vi "Process.vi"(8 "error in":errorcluster, 11 "DAQ":refnum<class "DAQ.lvclass">) -> (0 "error out":errorcluster, 3 "DAQ out":refnum<class "DAQ.lvclass">)   [LabVIEW 2019, in "DAQ.lvclass"]
doc: "---------------------------------------------------------------\nJKI State Machine Objects™\nhttp://jki.net/state-machine-objects/\nCopyright (C) 2005-2015, JKI <info@jki.net>\nALL RIGHTS RESERVED"
uses:
  DAQ.lvclass
  <vilib>/JKI/JKI SMO/SMO/SMO.lvclass
  <vilib>/JKI/JKI SMO/SMO/Typedefs/Parent Call--Enum.ctl
  Typedefs/PrivateEvents--DAQ.SetWaveform.ctl
  C:/Program Files (x86)/National Instruments/LabVIEW 2016/vi.lib/JKI/JKI SMO/SMO/SMO.lvclass
panel:
  out "Name":string
  # "DAQ process.vi"
  # "For instructions on how to use the JKI State Machine Objects, examples and video tutorials, visit:\nhttp://jki.net/state-machine-objects/\n\nJKI State Machine Objects™\nhttp://jki.net/state-machine-objects/\nCopyright (C) 2005-2015, JKI <info@jki.net>\nALL RIGHTS RESERVED"
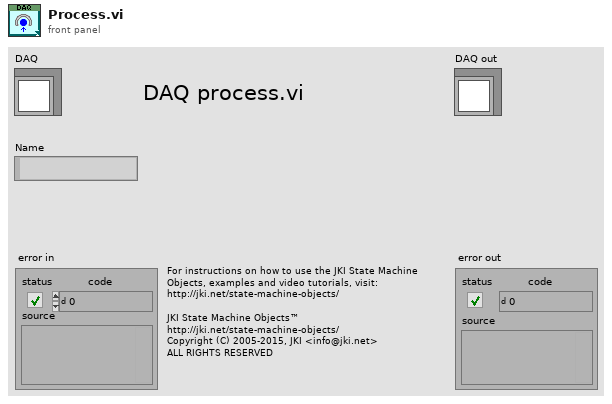
[diagram p1: front panel]
types:
  T1 = typedef "SMO.lvclass/Parent Call--Enum.ctl" = enum16{"Allows parent to run", "Does not request parent to run"}
  T2 = enum32{"invalid app kind", "Development System", "Run Time System", "Student Edition", "Embedded LabVIEW", "Evaluation", "Custom"}
  T3 = enum32{"Invalid", "Standard", "Closed", "Hidden", "Minimized", "Maximized"}
  T4 = enum32{"Bad", "Idle", "Run top level", "Running"}
  T5 = typedef "DAQ.lvclass/DAQ_Type.ctl" = enum16{"AI", "AO"}
  T6 = typedef "DAQ.lvclass/DAQ_SamplingInfo.ctl" = cluster{"Fs":dbl, "#s":i32}
  T7 = typedef "DAQ.lvclass/PrivateEvents--DAQ.SetWaveform.ctl" = waveform(dbl)[]
  T8 = cluster{"Core":cluster{"Current VI Reference":refnum<vi>, "Close Panel on Exit?":bool, "error":errorcluster}, "Self Reference":refnum<class "DAQ.lvclass">, "Channels":string, "DAQ_Type":T5, "DAQ_SamplingInfo":T6, "SetWaveform":T7, "to":i32}
  T9 = cluster{"Current VI Reference":refnum<vi>, "Close Panel on Exit?":bool, "error":errorcluster}
  T10 = typedef "SMO.lvclass/Protected Events.ctl" = cluster{"StopProcesses":refnum<user-event>, "AbortProcesses":refnum<user-event>, "Config Changed":refnum<user-event>, "Dependency":refnum<user-event>}
  T11 = typedef "DAQ.lvclass/PrivateEvents--Cluster.ctl" = cluster{"DAQ.Write":refnum<user-event>, "DAQ.setWaveform":refnum<user-event>}
  T12 = typedef "DAQ.lvclass/PrivateEvents--DAQ.Write.ctl" = waveform(dbl)[]
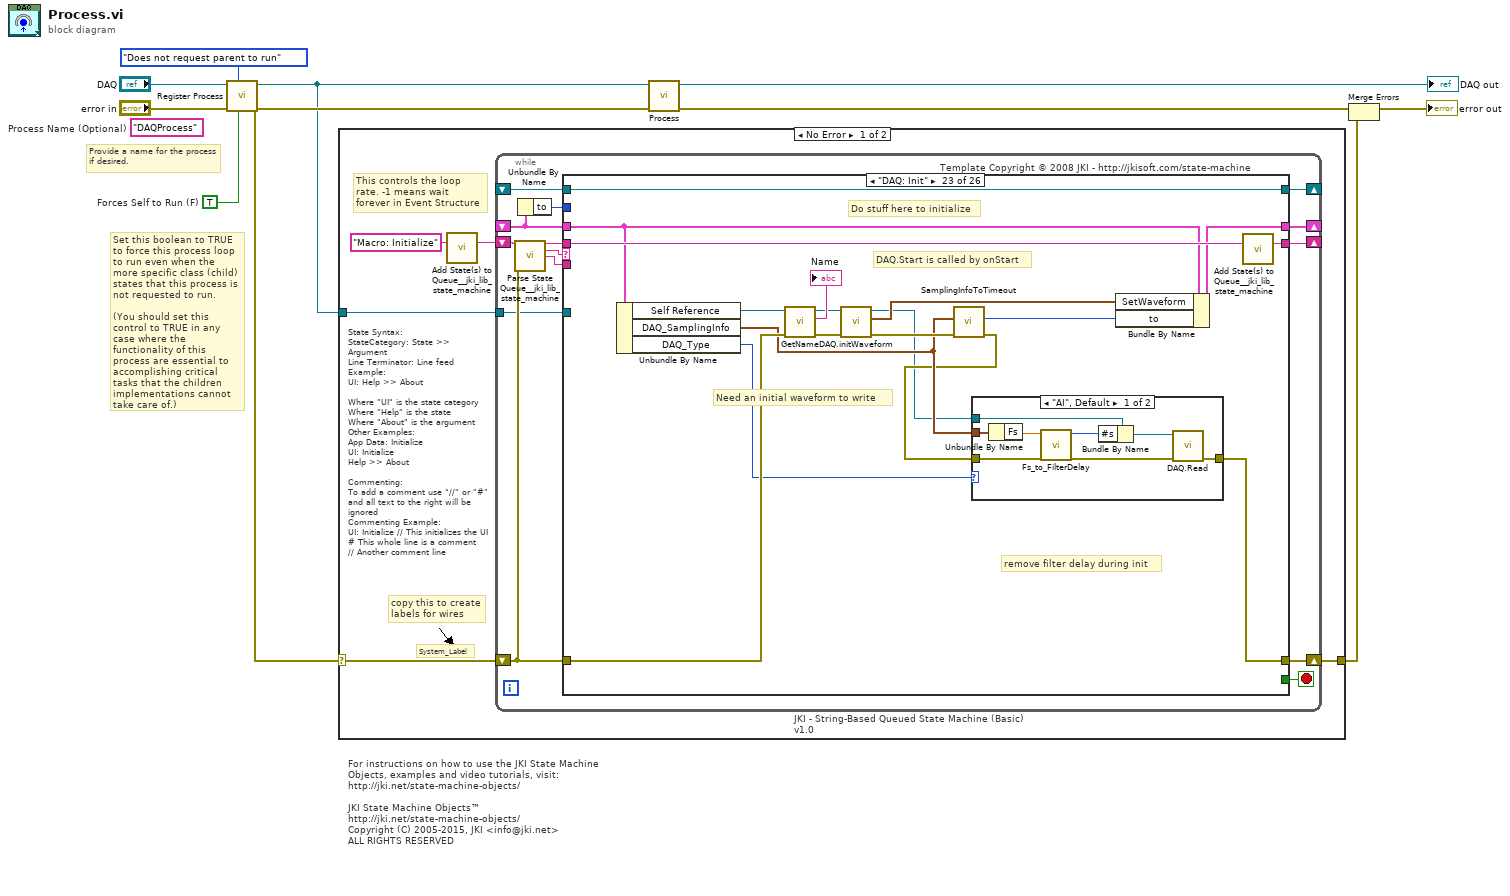
[diagram p0: block diagram]
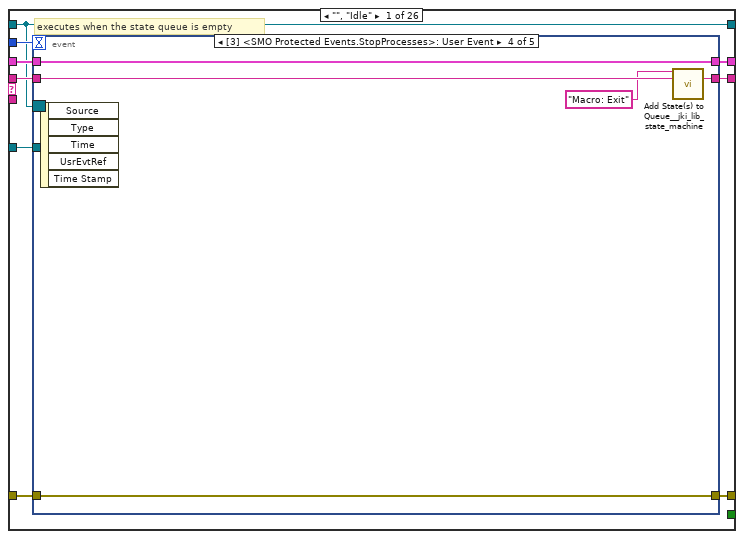
[diagram p2: hidden frame]
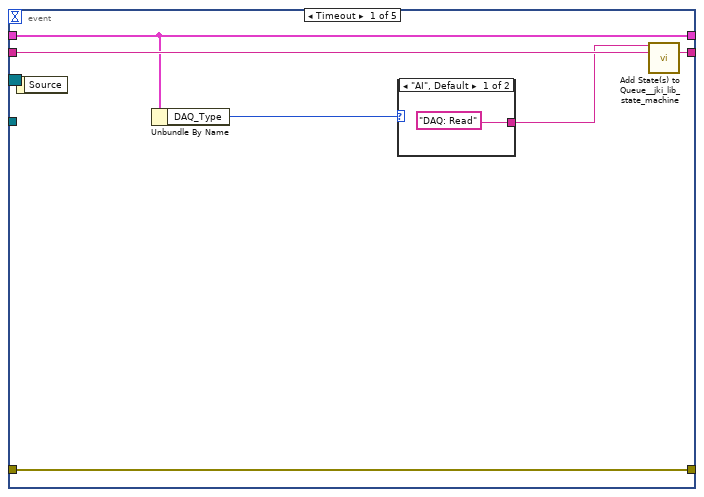
[diagram p3: hidden frame]
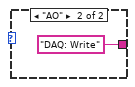
[diagram p4: hidden frame]
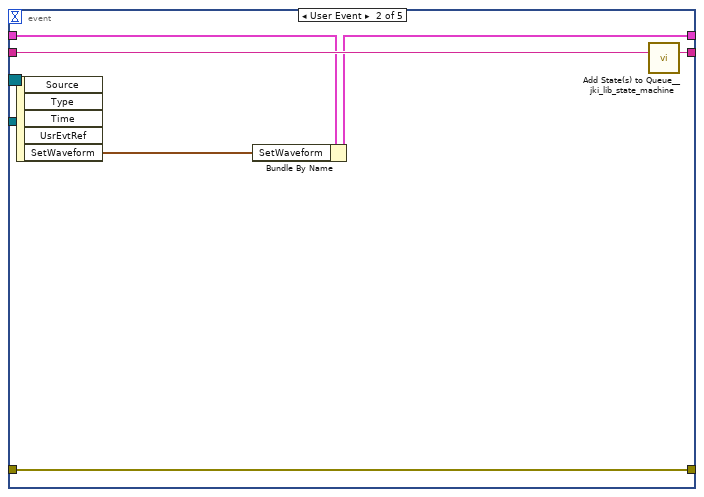
[diagram p5: hidden frame]
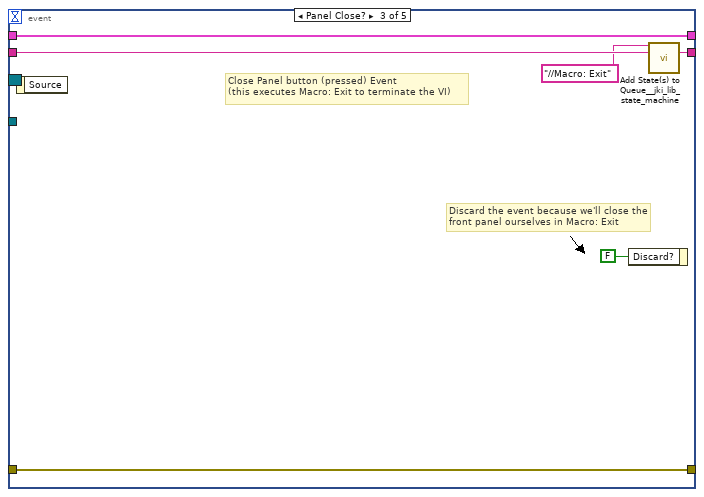
[diagram p6: hidden frame]
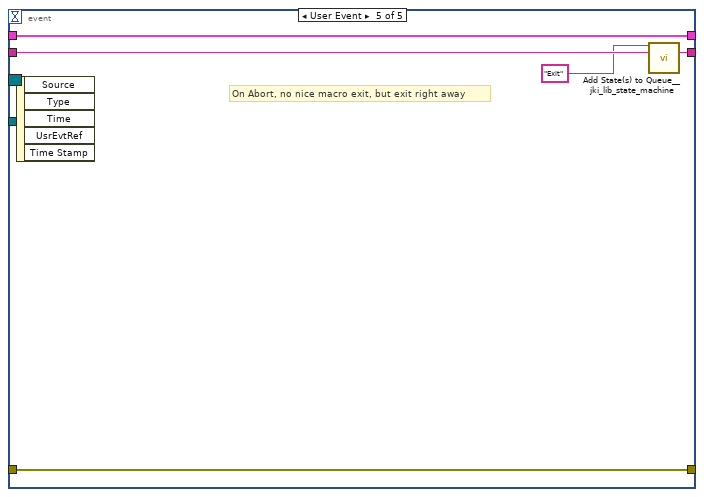
[diagram p7: hidden frame]
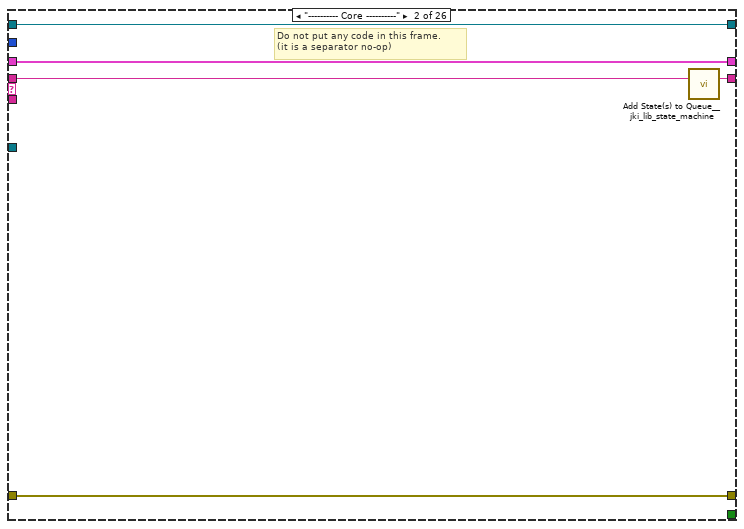
[diagram p8: hidden frame]
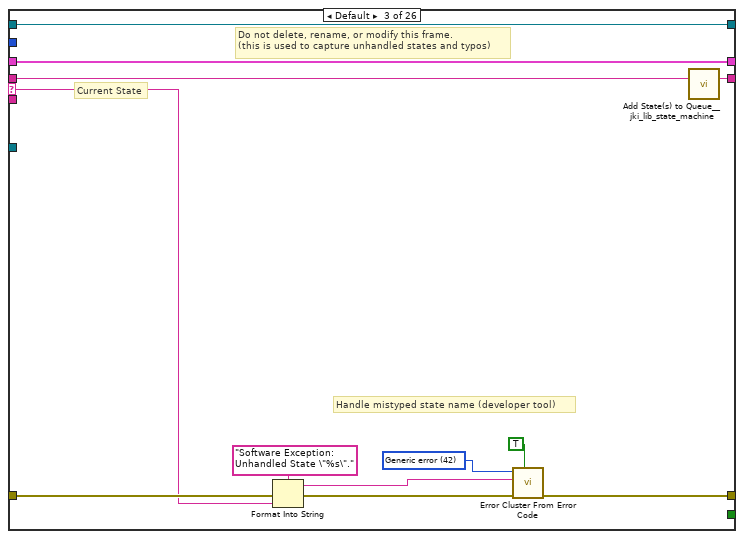
[diagram p9: hidden frame]
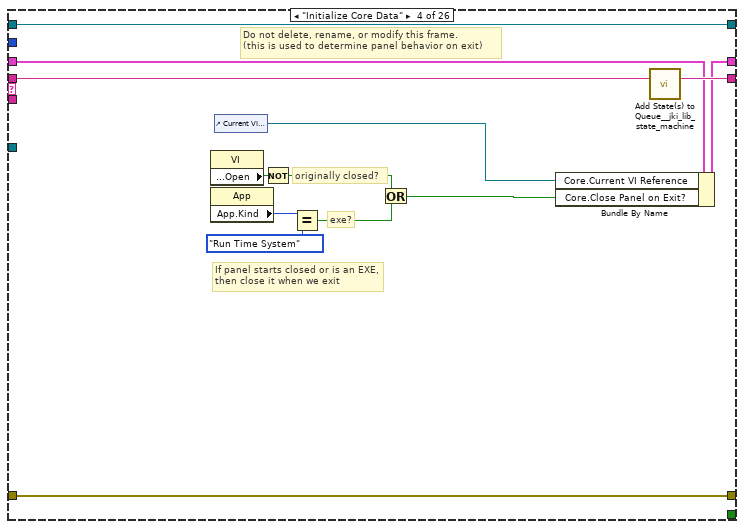
[diagram p10: hidden frame]
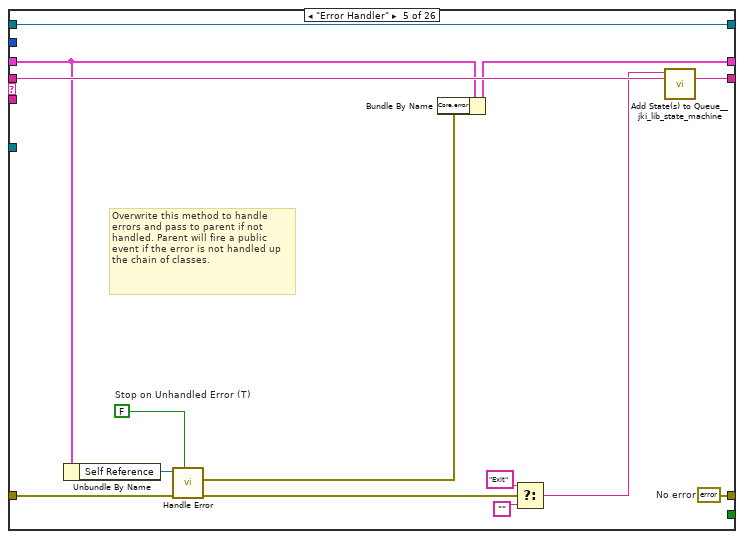
[diagram p11: hidden frame]
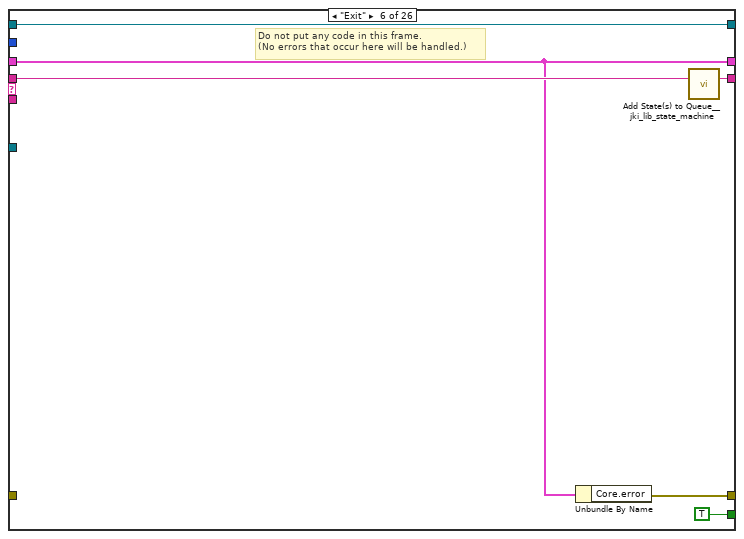
[diagram p12: hidden frame]
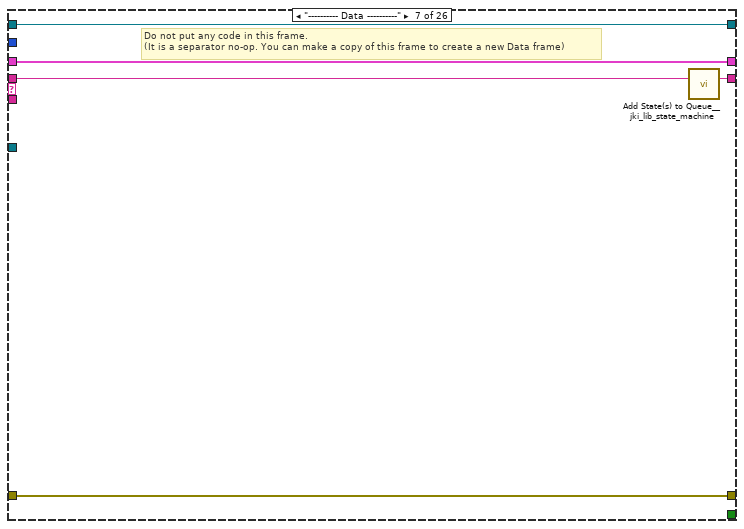
[diagram p13: hidden frame]
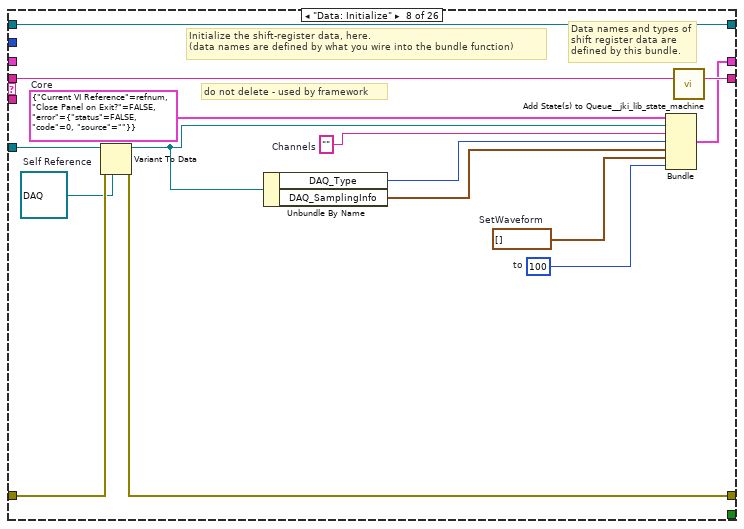
[diagram p14: hidden frame]
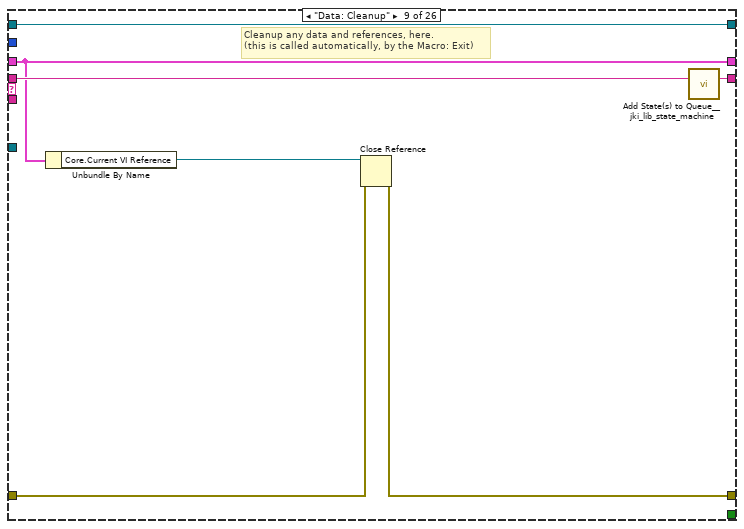
[diagram p15: hidden frame]
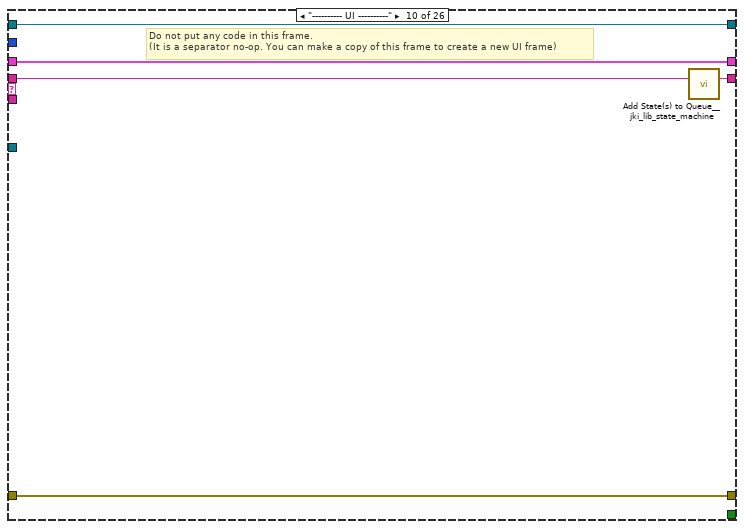
[diagram p16: hidden frame]
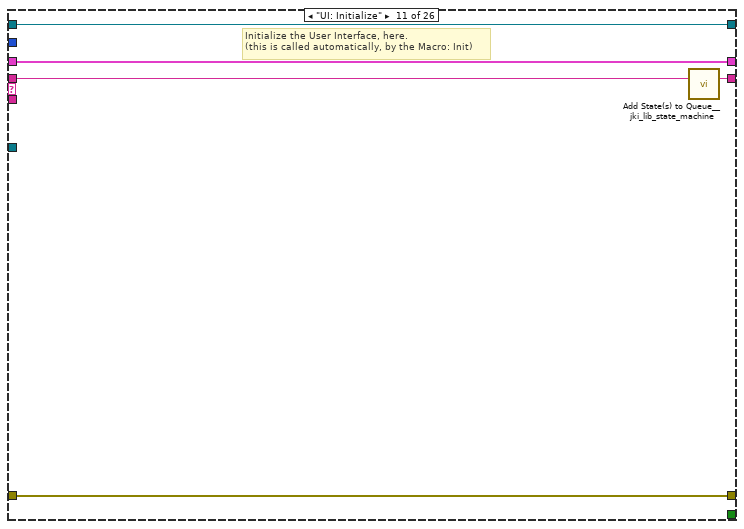
[diagram p17: hidden frame]
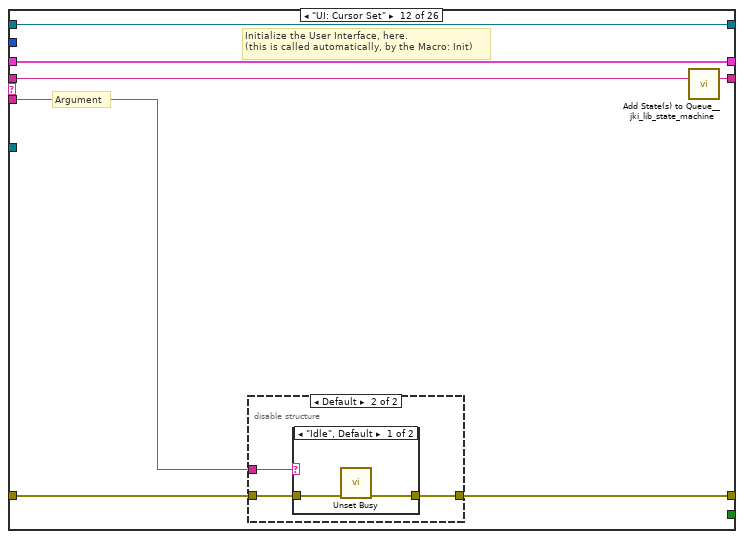
[diagram p18: hidden frame]
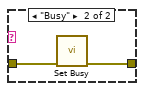
[diagram p20: hidden frame]
diagram:
  w1 = TRUE  # Forces Self to Run (F)
  (unwired) "DAQProcess"  # Process Name (Optional)
  # "Provide a name for the process\nif desired."
  # "Set this boolean to TRUE to force this process loop to run even when the more specific class (child) states that this process is not requested to run.\n\n(You should set this control to TRUE in any case where the functionality of this process are essential to accomplishing critical tasks that the children implementations cannot take care of.)"
  # "For instructions on how to use the JKI State Machine Objects, examples and video tutorials, visit:\nhttp://jki.net/state-machine-objects/\n\nJKI State Machine Objects™\nhttp://jki.net/state-machine-objects/\nCopyright (C) 2005-2015, JKI <info@jki.net>\nALL RIGHTS RESERVED"
  n1 = call <vilib>:"Register Process.vi"("Forces Self to Run (F)"=w1, "Parent Call"=Parent_Call--Enum."Does not request parent to run", "error in (no error)"="error in", "SMO"="DAQ") -> ("error out"=w7:errorcluster, "SMO out"=w6:refnum<class "DAQ.lvclass">)  [unwired: 6 in]
  n2 = case shown="No Error" w7 {
    selector: w7 -> [w12 w338]
    tunnel: w6 -> [w13 _]
    tunnel: [w11 w338] -> w3
    frame No Error {
      # "State Syntax:\nStateCategory: State >> Argument\nLine Terminator: Line feed\nExample:\nUI: Help >> About\n\nWhere \"UI\" is the state category\nWhere \"Help\" is the state\nWhere \"About\" is the argument\nOther Examples:\nApp Data: Initialize\nUI: Initialize\nHelp >> About\n\nCommenting:\nTo add a comment use \"//\" or \"#\" and all text to the right will be ignored\nCommenting Example:\nUI: Initialize // This initializes the UI\n# This whole line is a comment\n// Another comment line"
      # "copy this to create labels for wires"
      # "This controls the loop rate. -1 means wait forever in Event Structure"
      # "System_Label"
      n3 = call <vilib>:"Add State(s) to Queue__jki_lib_state_machine.vi"("State(s) in (\"\")"="Macro: Initialize") -> ("States Out"=w15:string)  [unwired: 14 in]
      n4 = while "JKI - String-Based Queued State Machine (Basic) v1.0" {
        shift-right: [w23] -> _
        shift-left: _ -> [w16]
        shift-right: [w18] -> w11
        shift-left: w12 -> [w22]
        shift-right: [w25] -> _
        shift-left: w15 -> [w26]
        tunnel: w13 -> [w21]
        shift-right: [w20] -> _
        shift-left: _ -> [w19]
        stop <- w24 stop-if-true
        # "Template Copyright © 2008 JKI - http://jkisoft.com/state-machine"
        n5 = call <vilib>:"Parse State Queue__jki_lib_state_machine.vi"("State Queue"=w26, "Error In (no error)"=w22) -> ("Remaining States"=w28:string, "Current State"=w29:string, "Arguments"=w27:string)  [unwired: 11 in]
        n6 = Unbundle By Name(w16) -> ("to"=w17:i32)
        n7 = case shown="\"DAQ: Init\"" w29 {
          selector: w29 -> [_ _ w75 _ _ _ _ _ _ _ _ _ _ _ _ _ _ _ _ _ _ _ _ _ _ _]
          tunnel: w28 -> [w38 w73 w79 w98 w112 w118 w123 w138 w145 w150 w155 w162 w180 w212 w226 w240 w245 w256 w261 w274 w280 w285 w303 w321 w332 w337]
          tunnel: w27 -> [_ _ _ _ _ _ _ _ _ _ _ w156 w175 _ _ _ _ _ _ _ _ _ _ _ _ _]
          tunnel: w16 -> [w36 w70 w77 w89 w106 w114 w120 _ w140 w147 w153 w160 w177 w209 w222 w231 w242 w253 w258 w272 w278 w283 w300 w312 w325 w333]
          tunnel: w22 -> [w34 w71 w80 w95 w108 _ w121 w134 w142 w148 w152 w158 w178 w210 w224 w238 w243 w248 w259 w268 w276 w281 w294 w314 w326 w334]
          tunnel: [w37 w72 w78 w97 w111 w117 w122 w137 w144 w149 w154 w161 w179 w211 w225 w239 w244 w255 w260 w273 w279 w284 w302 w320 w331 w336] -> w25
          tunnel: [_ _ _ _ _ TRUE _ _ _ _ _ _ _ _ _ _ _ _ _ _ _ _ _ _ _ _] -> w24
          tunnel: [w33 w70 w77 w96 w105 w114 w120 w136 w140 w147 w153 w160 w177 w209 w222 w231 w242 w253 w258 w272 w278 w283 w299 w312 w325 w333] -> w23
          tunnel: w17 -> [w32 _ _ _ _ _ _ _ _ _ _ _ _ _ _ _ _ _ _ _ _ _ _ _ _ _]
          tunnel: w21 -> [w30 _ _ _ _ _ _ w131 _ _ _ _ _ _ _ _ _ _ _ _ _ _ _ _ _ _]
          tunnel: [w31 w69 w74 w86 w110 w115 w119 w130 w139 w146 w151 w159 w174 w208 w223 w232 w241 w254 w257 w271 w277 w282 w301 w319 w330 w335] -> w20
          tunnel: w19 -> [w31 w69 w74 w86 w110 w115 w119 w130 w139 w146 w151 w159 w174 w208 w223 w232 w241 w254 w257 _ w277 w282 w301 w319 w330 w335]
          tunnel: [w35 w71 w81 w95 w107 w113 w121 w133 w141 w148 w152 w157 w172 w210 w224 w238 w243 w247 w259 w267 w276 w281 w286 w313 w324 w334] -> w18
          frame "", "Idle" {
            # "executes when the state queue is empty"
            n8 = event shown="[3] <SMO Protected Events.StopProcesses>: User Event" {
              selector: w31 -> [_ _ _ _ _]
              dyn-events: _ -> [_ _ _ _ _]
              timeout: w32 -> [_ _ _ _ _]
              tunnel: w38 -> [w44 w52 w58 w63 w68]
              tunnel: [w43 w51 w57 w62 w67] -> w37
              tunnel: w36 -> [w41 w49 w55 w60 w65]
              tunnel: [w42 w50 w56 w61 w66] -> w35
              tunnel: w34 -> [w42 w50 w56 w61 w66]
              tunnel: [w41 w48 w55 w60 w65] -> w33
              tunnel: w30 -> [_ _ _ _ _]
              event Timeout {
                n9 = event-data() -> ()  [unwired: 1 in, 1 out]
                n10 = Unbundle By Name(w41) -> ("DAQ_Type"=w40:T5)
                n11 = case shown="\"AI\", Default" w40 {
                  tunnel: ["DAQ: Read" ("State(s) at Back (\"\")") "DAQ: Write" ("State(s) at Back (\"\")")] -> w39
                  frame "AI", Default {
                  }
                  frame "AO" {
                  }
                }
                n12 = call <vilib>:"Add State(s) to Queue__jki_lib_state_machine.vi"("State(s) in Front (\"\")"=w39, "State(s) in (\"\")"=w44) -> ("States Out"=w43:string)  [unwired: 13 in]
              }
              event User Event {
                n13 = event-data() -> ("SetWaveform"=w47:waveform(dbl)[])  [unwired: 1 in, 4 out]
                n14 = Bundle By Name(cluster=w49, "SetWaveform"=w47) -> (w48:T8)
                n15 = call <vilib>:"Add State(s) to Queue__jki_lib_state_machine.vi"("State(s) in (\"\")"=w52) -> ("States Out"=w51:string)  [unwired: 14 in]
              }
              event Panel Close? {
                # "Discard the event because we'll close the front panel ourselves in Macro: Exit"
                # "Close Panel button (pressed) Event\n(this executes Macro: Exit to terminate the VI)"
                n16 = event-data() -> ()  [unwired: 1 in, 1 out]
                n17 = event-data("Discard?"=FALSE) -> ()  [unwired: 1 in, 1 out]
                n18 = call <vilib>:"Add State(s) to Queue__jki_lib_state_machine.vi"("State(s) in Front (\"\")"="//Macro: Exit", "State(s) in (\"\")"=w58) -> ("States Out"=w57:string)  [unwired: 13 in]
              }
              event User Event {
                n19 = event-data() -> ()  [unwired: 1 in, 5 out]
                n20 = call <vilib>:"Add State(s) to Queue__jki_lib_state_machine.vi"("State(s) in Front (\"\")"="Macro: Exit", "State(s) in (\"\")"=w63) -> ("States Out"=w62:string)  [unwired: 13 in]
              }
              event User Event {
                # "On Abort, no nice macro exit, but exit right away"
                n21 = event-data() -> ()  [unwired: 1 in, 5 out]
                n22 = call <vilib>:"Add State(s) to Queue__jki_lib_state_machine.vi"("State(s) in Front (\"\")"="Exit", "State(s) in (\"\")"=w68) -> ("States Out"=w67:string)  [unwired: 13 in]
              }
            }
          }
          frame "---------- Core ----------" {
            # "Do not put any code in this frame.\n(it is a separator no-op)"
            n23 = call <vilib>:"Add State(s) to Queue__jki_lib_state_machine.vi"("State(s) in (\"\")"=w73) -> ("States Out"=w72:string)  [unwired: 14 in]
          }
          frame Default {
            w84 = 42 items=["No error", "Argument error", "Memory is full", "Out of zone", "End of file", "File already open", "Generic file I/O error", "File not found", "File permission error", "Disk is full", "Duplicate path", "Too many files open", "System feature not enabled", "Resource file not found", "Cannot add resource", "Resource not found", "Image not found", "Image memory error", "Pen does not exist", "Config type invalid", "Config token not found", "Config parse error", "Config memory error", "Bad external code format", "Bad external code offset", "External code not present", "Null window", "Destroy window error", "Null menu", "Print aborted", "Bad print record", "Print driver error", "Windows error during printing", "Memory error during printing", "Print dialog error", "Generic print error", "Invalid device refnum", "Device not found", "Device parameter error", "Device unit error", "Cannot open device", "Device call aborted", "Generic error", "Cancelled by user", "Object ID too low", "Object ID too high", "Object not in heap", "Unknown heap", "Unknown object (invalid DefProc)", "Unknown object (DefProc not in table)", "Message out of range", "Invalid (null) method", "Unknown message", "Manager call not supported", "Bad address", "Network operation in progress", "Network operation timed out", "Connection is busy", "Network attribute not supported", "Network error", "Address in use", "System out of memory", "Connection aborted", "Connection refused", "Not connected", "Already connected", "Connection closed", "Initialization error (interapplication manager)", "Bad occurrence", "Wait on unbound occurrence handler", "Occurrence queue overflow", "Datalog type conflict", "Unused", "Unrecognized type (interapplication manager)", "Memory corrupt", "Failed to make temporary DLL", "Old CIN version", "Drag socket not found", "Failed to load drop-object", "Failed to register OLE object", "Failed to release OLE object", "Format specifier type mismatch", "Unknown format specifier", "Too few format specifiers", "Too many format specifiers", "Scan failed", "Newer CIN version", "Error converting to variant", "Runtime menu error", "Password tampered", "Variant attribute not found", "Incompatible variant data type", "Event data is not available", "Event Store is not present", "Occurrence is not found", "Event Queue is not created", "Event info is not available", "Refnum passed is NULL", "Error retrieving Class GUID", "Error retrieving CoClass GUID", "Error retrieving TypeLib GUID.", "Bad built application magic bytes.", "Specific driver is different from the specific driver associated with the Logical Name.", "There is no session opened to the class driver.", "Max Error", "MAX - Error with config objects", "MAX - Error loading configuration", "MAX - Group not supported"]
            # "Current State"
            # "Do not delete, rename, or modify this frame.\n(this is used to capture unhandled states and typos)"
            # "Handle mistyped state name (developer tool)"
            n24 = Format Into String(format string="Software Exception: Unhandled State \"%s\"." ("message"), error in=w80, w75) -> (resulting string=w83:string, error out=w82:errorcluster)  [unwired: 1 in]
            n25 = call <vilib>:"Error Cluster From Error Code.vi"("show call chain? (False)"=TRUE, "error in (no error)"=w82, "error message (\"\")"=w83, "error code (0)"=w84) -> ("error out"=w81:errorcluster)  [unwired: 5 in]
            n26 = call <vilib>:"Add State(s) to Queue__jki_lib_state_machine.vi"("State(s) in (\"\")"=w79) -> ("States Out"=w78:string)  [unwired: 14 in]
          }
          frame "Initialize Core Data" {
            # "Do not delete, rename, or modify this frame.\n(this is used to determine panel behavior on exit)"
            # "originally closed?"
            # "exe?"
            # "If panel starts closed or is an EXE, then close it when we exit"
            n27 = property class="VI"() -> ("Front Panel.Open"=w94:bool)  [unwired: 2 in, 2 out]
            n28 = property class="App"() -> ("App.Kind"=w93:T2)  [unwired: 2 in, 2 out]
            n29 = control-ref of="Current VI Reference"() -> (w87:refnum<vi>)
            n30 = Not(x=w94) -> (.not. x?=w91:bool)
            n31 = Equal?(x=w93, y=T2."Run Time System" ("Application:Kind")) -> (x = y?=w90:bool)
            n32 = Or(x=w91, y=w90) -> (x .or. y?=w88:bool)
            n33 = Bundle By Name(cluster=w89, "Core.Current VI Reference"=w87, "Core.Close Panel on Exit?"=w88) -> (w96:T8)
            n34 = call <vilib>:"Add State(s) to Queue__jki_lib_state_machine.vi"("State(s) in (\"\")"=w98) -> ("States Out"=w97:string)  [unwired: 14 in]
          }
          frame "Error Handler" {
            w99 = FALSE  # Stop on Unhandled Error (T)
            w107 = errorcluster {"status"=FALSE, "code"=0, "source"=""}  # No error
            # "Overwrite this method to handle errors and pass to parent if not handled. Parent will fire a public event if the error is not handled up the chain of classes."
            n35 = Unbundle By Name(w106) -> ("Self Reference"=w109:refnum<class "DAQ.lvclass">)
            n36 = call-dynamic "Handle Error.vi"("Stop on Unhandled Error (T)"=w99, "error in"=w108, "SMO"=w109) -> ("handling error"=w100:errorcluster, "Unhandled error"=w103:errorcluster)  [unwired: 6 in, 1 out]
            n37 = Bundle By Name(cluster=w106, "Core.error"=w103) -> (w105:T8)
            n38 = Select(t="Exit", s=w100, f="") -> (s? t:f=w104:string)
            n39 = call <vilib>:"Add State(s) to Queue__jki_lib_state_machine.vi"("State(s) in Front (\"\")"=w104, "State(s) in (\"\")"=w112) -> ("States Out"=w111:string)  [unwired: 13 in]
          }
          frame "Exit" {
            # "Do not put any code in this frame.\n(No errors that occur here will be handled.)"
            n40 = Unbundle By Name(w114) -> ("Core.error"=w113:errorcluster)
            n41 = call <vilib>:"Add State(s) to Queue__jki_lib_state_machine.vi"("State(s) in (\"\")"=w118) -> ("States Out"=w117:string)  [unwired: 14 in]
          }
          frame "---------- Data ----------" {
            # "Do not put any code in this frame.\n(It is a separator no-op. You can make a copy of this frame to create a new Data frame)"
            n42 = call <vilib>:"Add State(s) to Queue__jki_lib_state_machine.vi"("State(s) in (\"\")"=w123) -> ("States Out"=w122:string)  [unwired: 14 in]
          }
          frame "Data: Initialize" {
            w126 = 100  # to
            w125 = T7 []  # SetWaveform
            w129 = T9 {"Current VI Reference"=refnum, "Close Panel on Exit?"=FALSE, "error"={"status"=FALSE, "code"=0, "source"=""}}  # Core
            w132 = refnum<class "DAQ.lvclass"> refnum  # Self Reference
            w135 = ""  # Channels
            # "do not delete - used by framework"
            # "Data names and types of shift register data are defined by this bundle."
            # "Initialize the shift-register data, here.\n(data names are defined by what you wire into the bundle function)"
            n43 = Variant To Data(error in=w134, type=w132, Variant=w131) -> (data=w128:refnum<class "DAQ.lvclass">, error out=w133:errorcluster)
            n44 = Unbundle By Name(w128) -> ("DAQ_Type"=w127:T5, "DAQ_SamplingInfo"=w124:T6)
            n45 = Bundle("Core"=w129, "Self Reference"=w128, "Channels"=w135, "DAQ_Type"=w127, "DAQ_SamplingInfo"=w124, "SetWaveform"=w125, "to"=w126) -> (w136:T8)  [unwired: 1 in]
            n46 = call <vilib>:"Add State(s) to Queue__jki_lib_state_machine.vi"("State(s) in (\"\")"=w138) -> ("States Out"=w137:string)  [unwired: 14 in]
          }
          frame "Data: Cleanup" {
            # "Cleanup any data and references, here.\n(this is called automatically, by the Macro: Exit)"
            n47 = Unbundle By Name(w140) -> ("Core.Current VI Reference"=w143:refnum<vi>)
            n48 = Close Reference(reference=w143, error in (no error)=w142) -> (error out=w141:errorcluster)
            n49 = call <vilib>:"Add State(s) to Queue__jki_lib_state_machine.vi"("State(s) in (\"\")"=w145) -> ("States Out"=w144:string)  [unwired: 14 in]
          }
          frame "---------- UI ----------" {
            # "Do not put any code in this frame.\n(It is a separator no-op. You can make a copy of this frame to create a new UI frame)"
            n50 = call <vilib>:"Add State(s) to Queue__jki_lib_state_machine.vi"("State(s) in (\"\")"=w150) -> ("States Out"=w149:string)  [unwired: 14 in]
          }
          frame "UI: Initialize" {
            # "Initialize the User Interface, here.\n(this is called automatically, by the Macro: Init)"
            n51 = call <vilib>:"Add State(s) to Queue__jki_lib_state_machine.vi"("State(s) in (\"\")"=w155) -> ("States Out"=w154:string)  [unwired: 14 in]
          }
          frame "UI: Cursor Set" {
            # "Argument"
            # "Initialize the User Interface, here.\n(this is called automatically, by the Macro: Init)"
            n52 = disable-structure shown="Default" {
              disable-tunnel: w158 -> [w163 w166]
              disable-tunnel: [w163 w165] -> w157
              disable-tunnel: w156 -> [_ w164]
              frame condition #0 {
              }
              frame condition #1 (active) {
                n53 = case shown="\"Idle\", Default" w164 {
                  tunnel: w166 -> [w168 w170]
                  tunnel: [w167 w169] -> w165
                  frame "Idle", Default {
                    n54 = call <vilib>:"Unset Busy.vi"("error in (no error)"=w168) -> ("error out"=w167:errorcluster)  [unwired: 10 in]
                  }
                  frame "Busy" {
                    n55 = call <vilib>:"Set Busy.vi"("error in (no error)"=w170) -> ("error out"=w169:errorcluster)  [unwired: 9 in, 1 out]
                  }
                }
              }
            }
            n56 = call <vilib>:"Add State(s) to Queue__jki_lib_state_machine.vi"("State(s) in (\"\")"=w162) -> ("States Out"=w161:string)  [unwired: 14 in]
          }
          frame "UI: Front Panel State" {
            # "use for debugging"
            # "Argument"
            # "Set Front Panel Open or Closed\n(Usage: \"UI: Front Panel State >> Open|Close\")"
            n57 = Unbundle By Name(w177) -> ("Core.Current VI Reference"=w176:refnum<vi>)
            n58 = disable-structure shown="Default" {
              disable-tunnel: w178 -> [w184 w207]
              disable-tunnel: [w183 w207] -> w171
              disable-tunnel: w176 -> [w182 _]
              disable-tunnel: w175 -> [w181 _]
              frame condition #0 (active) {
                n59 = case shown="\"Close\"" w181 {
                  tunnel: w184 -> [w188 w201]
                  tunnel: [w190 w202] -> w183
                  tunnel: w182 -> [w189 w199]
                  frame "Open", Default {
                    n60 = property class="VI"(reference=w189, error in=w188) -> (reference out=w186:refnum<vi>, error out=w187:errorcluster, "FP.State"=w185:T3)
                    n61 = case shown="\"Closed\"" w185 {
                      tunnel: [w193 w196] -> w190
                      tunnel: w187 -> [w192 w196]
                      tunnel: w186 -> [w191 _]
                      frame "Closed" {
                        n62 = invoke class="VI" method="FP.Open"(reference=w191, error in=w192, "Activate"=TRUE, "State"=T3."Standard") -> (error out=w193:errorcluster)  [unwired: 1 in, 4 out]
                      }
                      frame Default {
                      }
                    }
                  }
                  frame "Close" {
                    n63 = property class="VI"(reference=w199, error in=w201) -> (reference out=w198:refnum<vi>, error out=w200:errorcluster, "FP.State"=w197:T3)
                    n64 = case shown="Default" w197 {
                      tunnel: [w203 w206] -> w202
                      tunnel: w200 -> [w203 w205]
                      tunnel: w198 -> [_ w204]
                      frame "Invalid", "Closed" {
                      }
                      frame Default {
                        n65 = invoke class="VI" method="FP.Close"(reference=w204, error in=w205) -> (error out=w206:errorcluster)  [unwired: 1 in, 2 out]
                      }
                    }
                  }
                }
              }
              frame condition #1 {
              }
            }
            n66 = call <userlib>:"Wait (ms)__ogtk.vi"("error in (no error)"=w171, "milliseconds to wait"=u32 0) -> ("error out"=w172:errorcluster)  [unwired: 8 in, 1 out]
            n67 = call <vilib>:"Add State(s) to Queue__jki_lib_state_machine.vi"("State(s) in (\"\")"=w180) -> ("States Out"=w179:string)  [unwired: 14 in]
          }
          frame "---------- Macro ----------" {
            # "Do not put any code in this frame.\n(It is a separator no-op. You can make a copy of this frame to create a new Macro frame)"
            n68 = call <vilib>:"Add State(s) to Queue__jki_lib_state_machine.vi"("State(s) in (\"\")"=w212) -> ("States Out"=w211:string)  [unwired: 14 in]
          }
          frame "Macro: Initialize" {
            w213 = "Process: Sync"
            w218 = "Data: Initialize\nInitialize Core Data\nUI: Initialize\nUI: Front Panel State >> Open\nEvents: Register"  # Data: Initialize Initialize Core Data UI: Initialize UI: Front Panel State >> Open Events: Register
            # "Initialization Macro\n(This is called once, when the VI starts)"
            n69 = control-ref of="This VI"() -> (w215:refnum<vi>)
            n70 = property class="VI"(reference=w215) -> ("Exec.State"=w214:T4)  [unwired: 1 in, 2 out]
            n71 = Equal?(x=w214, y=T4."Run top level") -> (x = y?=w220:bool)
            n72 = Select(t=w213, s=w220, f="") -> ()  [unwired: 1 out]
            n73 = call <vilib>:"Add State(s) to Queue__jki_lib_state_machine.vi"("State(s) in Front (\"\")"=w218, "State(s) in (\"\")"=w213, "State(s) at Back (\"\")"="DAQ: Init") -> ("States Out"=w216:string)  [unwired: 12 in]
            n74 = call <vilib>:"Add State(s) to Queue__jki_lib_state_machine.vi"("State(s) in Front (\"\")"=w216, "State(s) in (\"\")"=w226) -> ("States Out"=w225:string)  [unwired: 13 in]
          }
          frame "Macro: Exit" {
            # "Exit Macro\n(This is called once, when the VI exits)"
            n75 = Unbundle By Name(w231) -> ("Core.Close Panel on Exit?"=w237:bool)
            n76 = Select(t="DAQ: Stop\nUI: Front Panel State >> Close", s=w237, f="") -> (s? t:f=w234:string)
            n77 = call <vilib>:"Add State(s) to Queue__jki_lib_state_machine.vi"("State(s) in Front (\"\")"="Data: Cleanup\nEvents: Unregister", "State(s) in (\"\")"="Process: Sync", "State(s) at Back (\"\")"="Exit") -> ("States Out"=w228:string)  [unwired: 12 in]
            n78 = call <vilib>:"Add State(s) to Queue__jki_lib_state_machine.vi"("State(s) in (\"\")"=w234, "State(s) at Back (\"\")"=w228) -> ("States Out"=w233:string)  [unwired: 13 in]
            n79 = call <vilib>:"Add State(s) to Queue__jki_lib_state_machine.vi"("State(s) in Front (\"\")"=w233, "State(s) in (\"\")"=w240) -> ("States Out"=w239:string)  [unwired: 13 in]
          }
          frame "---------- Process ----------" {
            # "Template Separator\n(You can make a copy of, or modify, this frame)"
            n80 = call <vilib>:"Add State(s) to Queue__jki_lib_state_machine.vi"("State(s) in (\"\")"=w245) -> ("States Out"=w244:string)  [unwired: 14 in]
          }
          frame "Process: Sync" {
            n81 = Unbundle By Name(w253) -> ("Self Reference"=w249:refnum<class "DAQ.lvclass">)
            n82 = call <vilib>:"WaitOnProcessSync.vi"("error in (no error)"=w248, "SMO"=w249) -> ("error out"=w247:errorcluster, "Don't run?"=w252:bool)  [unwired: 7 in, 1 out]
            n83 = Select(t="Data: Cleanup\nEvents: Unregister\nExit", s=w252, f="") -> (s? t:f=w246:string)
            n84 = call <vilib>:"Add State(s) to Queue__jki_lib_state_machine.vi"("State(s) in Front (\"\")"=w246, "State(s) in (\"\")"=w256) -> ("States Out"=w255:string)  [unwired: 13 in]
          }
          frame "---------- Events ----------" {
            # "Template Separator\n(You can make a copy of, or modify, this frame)"
            n85 = call <vilib>:"Add State(s) to Queue__jki_lib_state_machine.vi"("State(s) in (\"\")"=w261) -> ("States Out"=w260:string)  [unwired: 14 in]
          }
          frame "Events: Register" {
            # "Expand to add\nmore events"
            n86 = Unbundle By Name(w272) -> ("Self Reference"=w269:refnum<class "DAQ.lvclass">)
            n87 = call <vilib>:"GetProtectedEvents.vi"("SMO"=w269) -> ("error out"=w265:errorcluster, "SMO Protected Events"=w270:T10, "SMO out"=w262:refnum<class "DAQ.lvclass">)  [unwired: 8 in]
            n88 = call "DAQ.GetPrivateEvents.vi"("DAQ"=w262) -> ("error out"=w264:errorcluster, "Private Events"=w263:T11)  [unwired: 8 in, 1 out]
            n89 = register-events(w270, w263) -> (reference out=w271:refnum<event-registration>, error out=w266:errorcluster)  [unwired: 2 in]
            n90 = Merge Errors(w268, w266, w265, w264) -> (w267:errorcluster)
            n91 = call <vilib>:"Add State(s) to Queue__jki_lib_state_machine.vi"("State(s) in (\"\")"=w274) -> ("States Out"=w273:string)  [unwired: 14 in]
          }
          frame "Events: Unregister" {
            n92 = Unregister For Events(event registration refnum=w277, error in=w276) -> (error out=w275:errorcluster)
            n93 = call <vilib>:"Clear Errors.vi"("error in (no error)"=w275) -> ()  [unwired: 5 in, 2 out]
            n94 = call <vilib>:"Add State(s) to Queue__jki_lib_state_machine.vi"("State(s) in (\"\")"=w280) -> ("States Out"=w279:string)  [unwired: 14 in]
          }
          frame "---------- Action ----------" {
            n95 = call <vilib>:"Add State(s) to Queue__jki_lib_state_machine.vi"("State(s) in (\"\")"=w285) -> ("States Out"=w284:string)  [unwired: 14 in]
          }
          frame "DAQ: Init" {
            # "remove filter delay during init"
            # "Need an initial waveform to write"
            # "DAQ.Start is called by onStart"
            # "Do stuff here to initialize"
            n96 = Unbundle By Name(w300) -> ("Self Reference"=w297:refnum<class "DAQ.lvclass">, "DAQ_SamplingInfo"=w290:T6, "DAQ_Type"=w288:T5)
            n97 = call <vilib>:"GetName.vi"("error in (no error)"=w294, "SMO"=w297) -> ("error out"=w295:errorcluster, "Name"=→"Name":string, "SMO out"=w296:refnum<class "DAQ.lvclass">)  [unwired: 6 in, 1 out]
            n98 = call "DAQ.initWaveform.vi"("error in (no error)"=w295, "DAQ in"=w296) -> ("error out"=w292:errorcluster, "Waveforms"=w291:waveform(dbl)[], "DAQ out"=w287:refnum<class "DAQ.lvclass">)  [unwired: 7 in]
            n99 = call "SamplingInfoToTimeout.vi"("error in"=w292, "sampling info"=w290) -> ("error out"=w289:errorcluster, "timeout (ms)"=w293:i32)  [unwired: 7 in]
            n100 = case shown="\"AI\", Default" w288 {
              tunnel: w290 -> [w310 _]
              tunnel: w287 -> [w304 _]
              tunnel: [w306 w311] -> w286
              tunnel: w289 -> [w305 w311]
              frame "AI", Default {
                n101 = Unbundle By Name(w310) -> ("Fs"=w309:dbl)
                n102 = call "Fs_to_FilterDelay.vi"("Fs"=w309) -> ("Total Filter Delay (samples)"=w308:u32)  [unwired: 10 in]
                n103 = Bundle By Name(cluster=w304, "#s"=w308) -> (w307:refnum<class "DAQ.lvclass">)
                n104 = call-dynamic "DAQ.Read.vi"("error in (no error)"=w305, "DAQ in"=w307) -> ("error out"=w306:errorcluster)  [unwired: 7 in, 2 out]
              }
              frame "AO" {
              }
            }
            n105 = Bundle By Name(cluster=w300, "SetWaveform"=w291, "to"=w293) -> (w299:T8)
            n106 = call <vilib>:"Add State(s) to Queue__jki_lib_state_machine.vi"("State(s) in (\"\")"=w303) -> ("States Out"=w302:string)  [unwired: 14 in]
          }
          frame "DAQ: Read" {
            # "why not put inside DAQ.Read?"
            # "fire event"
            # "read wfm from DAQ"
            n107 = Unbundle By Name(w312) -> ("Self Reference"=w316:refnum<class "DAQ.lvclass">)
            n108 = call-dynamic "DAQ.Read.vi"("error in (no error)"=w314, "DAQ in"=w316) -> ("error out"=w317:errorcluster, "Read"=w315:waveform(dbl)[], "DAQ out"=w318:refnum<class "DAQ.lvclass">)  [unwired: 7 in]
            n109 = call "DAQ.Read.PrivateEvent.vi"("error in (no error)"=w317, "DAQ.Read"=w315, "DAQ"=w318) -> ("error out"=w313:errorcluster)  [unwired: 7 in, 1 out]
            n110 = call <vilib>:"Add State(s) to Queue__jki_lib_state_machine.vi"("State(s) in (\"\")"=w321) -> ("States Out"=w320:string)  [unwired: 14 in]
          }
          frame "DAQ: Write" {
            # "why not put in DAQ.Write?"
            # "fire event with write wfm"
            # "write wfm to DAQ"
            n111 = Unbundle By Name(w325) -> ("SetWaveform"=w323:T7, "Self Reference"=w327:refnum<class "DAQ.lvclass">)
            n112 = call-dynamic "DAQ.Write.vi"("error in (no error)"=w326, "Write"=w323, "DAQ in"=w327) -> ("error out"=w329:errorcluster, "Written Waveform"=w322:T12, "DAQ out"=w328:refnum<class "DAQ.lvclass">)  [unwired: 6 in]
            n113 = call "DAQ.Write.PrivateEvent.vi"("error in (no error)"=w329, "DAQ.Write"=w322, "DAQ"=w328) -> ("error out"=w324:errorcluster)  [unwired: 7 in, 1 out]
            n114 = call <vilib>:"Add State(s) to Queue__jki_lib_state_machine.vi"("State(s) in (\"\")"=w332) -> ("States Out"=w331:string)  [unwired: 14 in]
          }
          frame "DAQ: Stop" {
            # "DAQ.Stop is called by onStop.vi\nDAQ.Clear is called by onDestroy.vi"
            n115 = call <vilib>:"Add State(s) to Queue__jki_lib_state_machine.vi"("State(s) in (\"\")"=w337) -> ("States Out"=w336:string)  [unwired: 14 in]
          }
        }
      }
    }
    frame Error {
    }
  }
  n116 = call-parent "Process.vi"("error in"=w7, "SMO"=w6) -> ("error out"=w4:errorcluster, "SMO out"=→"DAQ out":refnum<class "DAQ.lvclass">)  [unwired: 8 in]
  n117 = Merge Errors(w4, w3) -> (→"error out":errorcluster)
